vi "Actor Core.vi"(8 "error in":errorcluster, 11 "Chat Window Model in":refnum<class "Chat Window Model.lvclass">) -> (0 "error out":errorcluster, 3 "Actor out":refnum<class "Actor.lvclass">)   [LabVIEW 2020, in "Chat Window Model.lvlib" / "Chat Window Model.lvclass"]
doc: "(<B>Filename</B>: Actor Framework.lvlib:Actor.lvclass:Actor Core.vi)\n\nReceives messages to the actor, reacts to them, and initiates any error handling that may shut the actor down.\n\nDescendant classes may override this VI to append parallel tasks for the actor to complete while it handles messages. Overrides use the Call Parent Method node."
uses:
  Chat Window Model.lvclass
  C:/Program Files/National Instruments/LabVIEW 2020/vi.lib/ActorFramework/Actor/Actor.lvclass
  <vilib>/ActorFramework/Actor/Actor.lvclass
  Chat Window Interface/Chat Window Interface/Chat Window Interface.lvclass
  C:/Users/huipeng8/Desktop/Chat-Window-Tutorial-Series/LabVIEW Interfaces/Chat Window UI Controller/Chat Window UI Controller/Chat Window UI Controller.lvclass
  Chat Window Model.lvclass/Chat Window Model.ctl
  Chat Window UI Controller/Chat Window UI Controller/Chat Window UI Controller.lvclass/Chat Window UI Controller.ctl
  <vilib>/ActorFramework/Actor/Actor.lvclass/Actor.ctl
  <vilib>/ActorFramework/Message Enqueuer/Message Enqueuer.lvclass/Message Enqueuer.ctl
  SubPanel-Actor-Framework-master/Event-Source-Actor/Source/Template Source/Event Source Messages/Register For Event Msg/Register For Event Msg.lvclass/Register For Event Msg.ctl
  <vilib>/ActorFramework/Message Enqueuer/Init from Existing Queue.vi
  <vilib>/ActorFramework/Message Enqueuer/Enqueue.vi
  SubPanel-Actor-Framework-master/Event-Source-Actor/Source/Template Source/Event Source Messages/Register For Event Msg/Register For Event Msg.lvclass
  C:/Program Files/National Instruments/LabVIEW 2020/vi.lib/ActorFramework/Message/Message.lvclass
  <vilib>/ActorFramework/Message Priority Queue/Priority Enqueue.vi
  <vilib>/ActorFramework/Message Enqueuer/Message Enqueuer.lvclass
  SubPanel-Actor-Framework-master/Event-Source-Actor/Source/Template Source/Event Source Actor/Event Source Actor.lvclass
  Chat Window UI Controller/Chat Window UI Controller/Chat Window UI Controller.lvclass
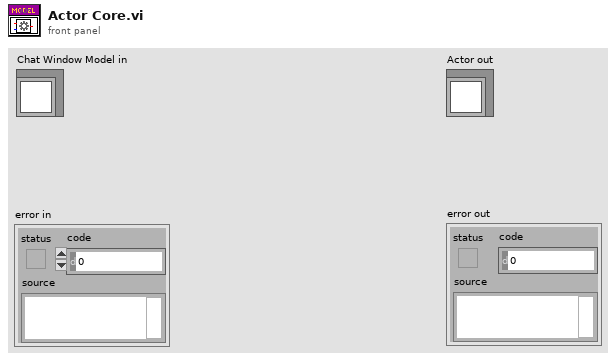
[diagram p1: front panel]
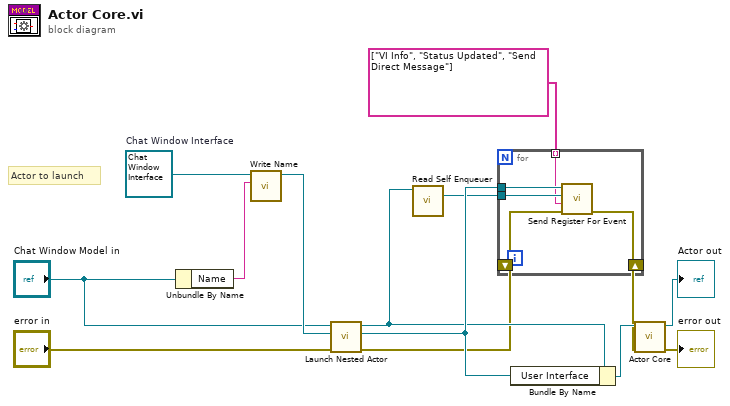
[diagram p0: block diagram]
diagram:
  w7 = refnum<class "Chat Window Interface.lvclass"> refnum  # Chat Window Interface
  # "Actor to launch"
  n1 = Unbundle By Name("Chat Window Model in") -> ("Name"=w8:string)
  n2 = call "Write Name.vi"("Name"=w8, "Chat Window UI Controller in"=w7) -> ("Chat Window UI Controller out"=w10:refnum<class "Chat Window Interface.lvclass">)  [unwired: 8 in, 1 out]
  n3 = call <vilib>:"Launch Nested Actor.vi"("error in (no error)"="error in", "Nested Actor"=w10, "Caller Actor in"="Chat Window Model in") -> ("error out"=w3:errorcluster, "Nested Actor's Enqueuer"=w6:refnum<class "Message Enqueuer.lvclass">, "Caller Actor out"=w5:refnum<class "Chat Window Model.lvclass">)  [unwired: 6 in]
  n4 = call <vilib>:"Read Self Enqueuer.vi"("Actor"=w5) -> ("Self Enqueuer"=w4:refnum<class "Message Enqueuer.lvclass">)  [unwired: 10 in]
  n5 = for {
    tunnel: w6 -> [w19]
    tunnel: w4 -> [w18]
    shift-right: [w16] -> w2
    shift-left: w3 -> [w17]
    tunnel: string[] ["VI Info", "Status Updated", "Send Direct Message"] -> [w15] mode=indexing
    n6 = call "Send Register For Event.vi"("error in"=w17, "Event Name"=w15, "Registrant Enq"=w18, "Message Enqueuer"=w19) -> ("error out"=w16:errorcluster)  [unwired: 6 in, 1 out]
  }
  n7 = Bundle By Name(cluster=w5, "User Interface"=w6) -> (w11:refnum<class "Chat Window Model.lvclass">)
  n8 = call-parent "Actor Core.vi"("error in"=w2, "Actor in"=w11) -> ("error out"=→"error out":errorcluster, "Actor out"=→"Actor out":refnum<class "Actor.lvclass">)  [unwired: 8 in]
